vi "json Parse Path - string path.vi"(8 "error in (no error)":errorcluster, 9 "default":path, 10 "path":string, 11 "JSON Document in":refnum<class "JSON Document.lvclass">) -> (0 "error out":errorcluster, 1 "defaulted?":bool, 2 "value":path, 3 "JSON Document out":refnum<class "JSON Document.lvclass">)   [LabVIEW 2015, in "JSON Document.lvclass"]
uses:
  JSON Document.lvclass
  json Parse String - string path.vi
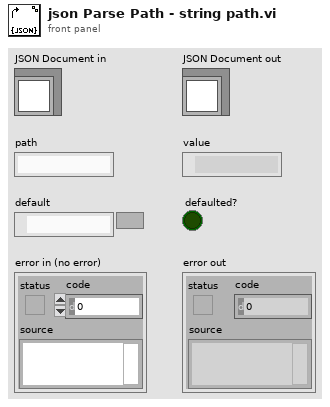
[diagram p1: front panel]
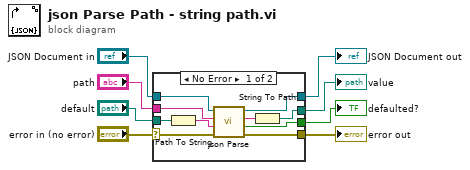
[diagram p0: block diagram]
diagram:
  n1 = case shown="No Error" "error in (no error)" {
    selector: "error in (no error)" -> [w16 w21]
    tunnel: [w15 w21] -> w7
    tunnel: [w9 w20] -> w5
    tunnel: "JSON Document in" -> [w10 w20]
    tunnel: "default" -> [w18 w19]
    tunnel: "path" -> [w17 _]
    tunnel: [w14 w19] -> w2
    tunnel: [w13 _] -> w1
    frame No Error {
      n2 = Path To String(path=w18) -> (string=w12:string)
      n3 = call-poly "json Parse.vi"("error in (no error)"=w16, "default"=w12, "path"=w17, "JSON Document in"=w10) -> ("error out"=w15:errorcluster, "defaulted?"=w13:bool, "value"=w11:string, "JSON Document out"=w9:refnum<class "JSON Document.lvclass">)  [unwired: 4 in]
      n4 = String To Path(string=w11) -> (path=w14:path)
    }
    frame Error {
    }
  }
  "error out" <- w7
  "JSON Document out" <- w5
  "value" <- w2
  "defaulted?" <- w1
